vi "StripXMLNS.vi"(1 "XML in":string) -> (0 "XML out":string)   [LabVIEW 2013, in "SetListPrefs.lvclass"]
uses:
  SetListPrefs.lvclass
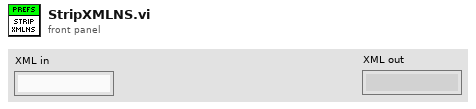
[diagram p1: front panel]
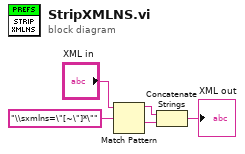
[diagram p0: block diagram]
diagram:
  n1 = Match Pattern(string="XML in", regular expression="\\sxmlns=\"[~\"]*\"") -> (before substring=w4:string, after substring=w5:string)  [unwired: 1 in, 2 out]
  n2 = Concatenate Strings(w4, w5) -> (→"XML out":string)
